vi "Splash Screen Launch Tester.vi"   [LabVIEW 2020]
panel:
  # "Run Me"
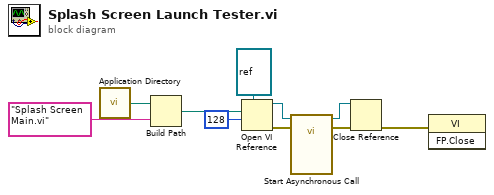
[diagram p0: block diagram]
diagram:
  n1 = call <vilib>:"Application Directory.vi"() -> ("Application Directory"=w6:path)
  n2 = Build Path(base path=w6, name or relative path="Splash Screen Main.vi") -> (appended path=w4:path)
  n3 = Open VI Reference(type specifier VI Refnum (for type only)=refnum<vi> refnum, vi path=w4, options=128) -> (vi reference=w9:refnum<vi>, error out=w10:errorcluster)  [unwired: 3 in]
  n4 = call-by-ref "Start Asynchronous Call"(reference=w9, error in=w10) -> (reference out=w2:refnum<vi>, error out=w3:errorcluster)  [unwired: 12 in]
  n5 = Close Reference(reference=w2, error in (no error)=w3) -> (error out=w1:errorcluster)
  n6 = invoke class="VI" method="FP.Close"(error in=w1) -> ()  [unwired: 2 in, 3 out]
